vi "Dialog Title.vi"(11 "Action":T1=enum."Wire Properties") -> (3 "Window Title":string)   [LabVIEW 2023]
uses:
  controls/action enum.ctl
  controls/action_menu text cluster.ctl
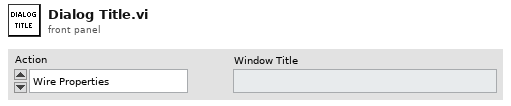
[diagram p1: front panel]
types:
  T1 = typedef "action enum.ctl" = enum16{"[NONE]", "APP_SEPARATOR", "Wire Bundle", "Wire Unbundle", "Terminal Unbundle", "Terminal Bundle", "Bundler Move Up", "Bundler Move Down", "Bundler Insert", "Bundler Remove", "Bundler Remove Unwired", "Bundler Reorder", "In Place Insert", "In Place Remove", "In Place Remove Unwired", "In Place Reorder", "Wire Properties", "Wire Method", "Terminal Properties", "Terminal Method", "Property Move Up", "Property Move Down", "Properties Insert", "Properties Remove", "Properties Remove Unwired", "Properties Reorder", "Method Change", "Class For Constant", "Class For Control", "Class For Node", "Class Name to Clipboard"}
  T2 = typedef "action_menu text cluster.ctl" = cluster{"Action":T1, "Window Title":string}
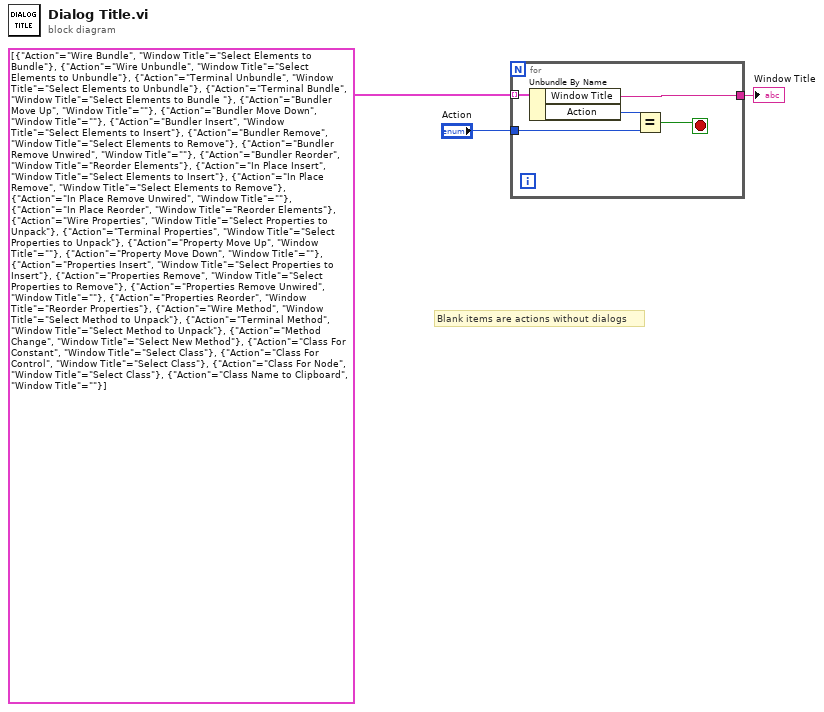
[diagram p0: block diagram]
diagram:
  # "Blank items are actions without dialogs"
  n1 = for {
    tunnel: T2[] [{"Action"=enum."Wire Bundle", "Window Title"="Select Elements to Bundle"}, {"Action"=enum."Wire Unbundle", "Window Title"="Select Elements to Unbundle"}, {"Action"=enum."Terminal Unbundle", "Window Title"="Select Elements to Unbundle"}, {"Action"=enum."Terminal Bundle", "Window Title"="Select Elements to Bundle "}, {"Action"=enum."Bundler Move Up", "Window Title"=""}, {"Action"=enum."Bundler Move Down", "Window Title"=""}, {"Action"=enum."Bundler Insert", "Window Title"="Select Elements to Insert"}, {"Action"=enum."Bundler Remove", "Window Title"="Select Elements to Remove"}, {"Action"=enum."Bundler Remove Unwired", "Window Title"=""}, {"Action"=enum."Bundler Reorder", "Window Title"="Reorder Elements"}, {"Action"=enum."In Place Insert", "Window Title"="Select Elements to Insert"}, {"Action"=enum."In Place Remove", "Window Title"="Select Elements to Remove"}, {"Action"=enum."In Place Remove Unwired", "Window Title"=""}, {"Action"=enum."In Place Reorder", "Window Title"="Reorder Elements"}, {"Action"=enum."Wire Properties", "Window Title"="Select Properties to Unpack"}, {"Action"=enum."Terminal Properties", "Window Title"="Select Properties to Unpack"}, {"Action"=enum."Property Move Up", "Window Title"=""}, {"Action"=enum."Property Move Down", "Window Title"=""}, {"Action"=enum."Properties Insert", "Window Title"="Select Properties to Insert"}, {"Action"=enum."Properties Remove", "Window Title"="Select Properties to Remove"}, {"Action"=enum."Properties Remove Unwired", "Window Title"=""}, {"Action"=enum."Properties Reorder", "Window Title"="Reorder Properties"}, {"Action"=enum."Wire Method", "Window Title"="Select Method to Unpack"}, {"Action"=enum."Terminal Method", "Window Title"="Select Method to Unpack"}, {"Action"=enum."Method Change", "Window Title"="Select New Method"}, {"Action"=enum."Class For Constant", "Window Title"="Select Class"}, {"Action"=enum."Class For Control", "Window Title"="Select Class"}, {"Action"=enum."Class For Node", "Window Title"="Select Class"}, {"Action"=enum."Class Name to Clipboard", "Window Title"=""}] -> [w8] mode=indexing
    tunnel: "Action" -> [w6]
    tunnel: [w5] -> w1
    stop <- w4 stop-if-true
    n2 = Unbundle By Name(w8) -> ("Window Title"=w5:string, "Action"=w7:T1)
    n3 = Equal?(x=w7, y=w6) -> (x = y?=w4:bool)
  }
  "Window Title" <- w1
